vi "周期设置.vi"(11 "定时控制参数输入":T1) -> (3 "定时控制参数输出":T1)   [LabVIEW 2016, in "质控单元.lvlib"]
uses:
  <vilib>/Utility/miscctls.llb/LVPointTypeDef.ctl
panel:
  in  "采配水启用":bool
  in  "模块选择":T2
  in  "确定":bool
  in  "取消":bool
  in  "定时功能启用":bool
  out "选项卡控件":enum32{"定点启动", "间隔启动"}(tab)
  in  "24H周期设置":bool[](xcontrol)
  in  "已经启动次数":dbl
  in  "设定启动次数":dbl
  in  "定时间隔":dbl
  in  "周期设置类型":enum16{"定点启动", "间隔启动"}(ring)
  # "仪器测试类型："
  # "周期设置类型："
  # "请输入定时启动间隔"
  # "min"
  # "次"
  # "次"
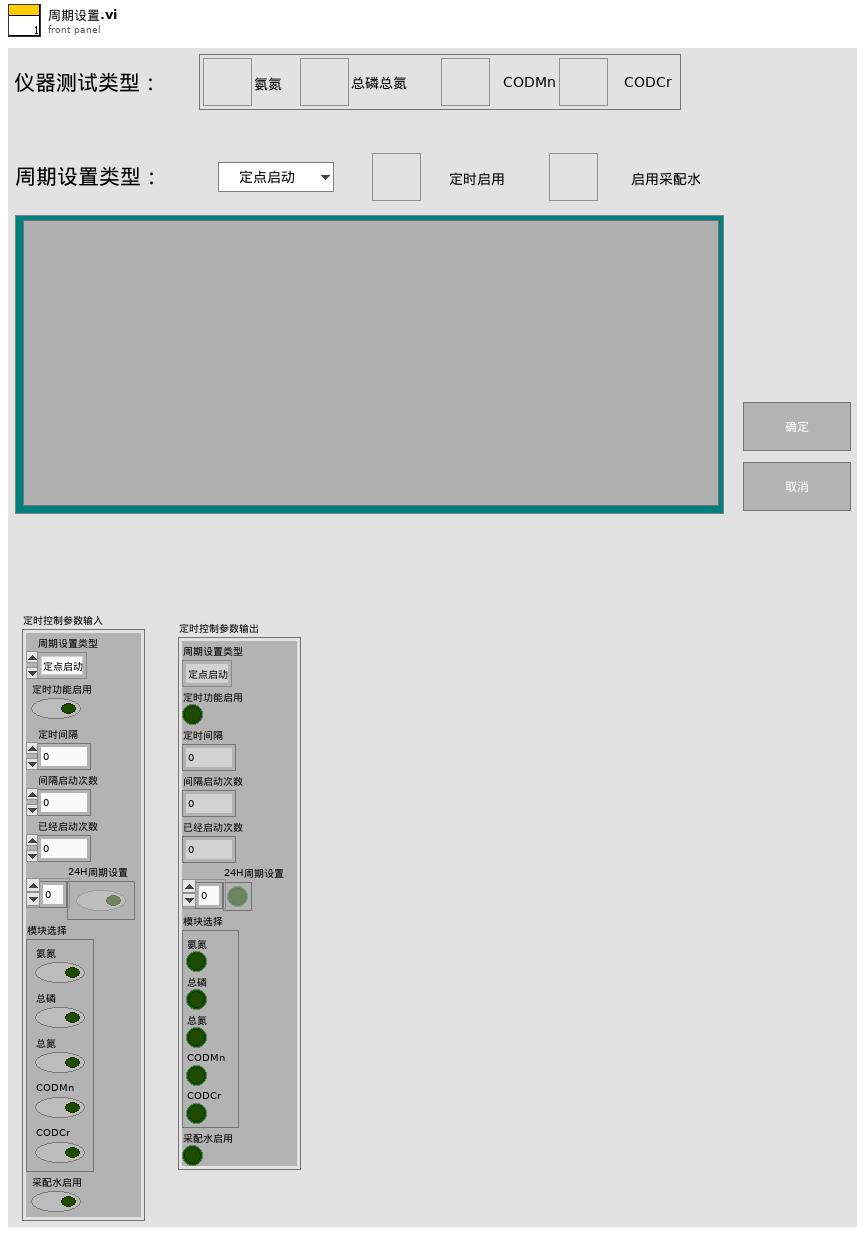
[diagram p1: front panel]
types:
  T1 = cluster{"周期设置类型":enum16{"定点启动", "间隔启动"}, "定时功能启用":bool, "定时间隔":dbl, "间隔启动次数":dbl, "已经启动次数":dbl, "24H周期设置":bool[], "模块选择":cluster{"氨氮":bool, "总磷":bool, "总氮":bool, "CODMn":bool, "CODCr":bool}, "采配水启用":bool}
  T2 = cluster{"氨氮":bool, "总磷":bool, "总氮":bool, "CODMn":bool, "CODCr":bool}
  T3 = typedef "LVPointTypeDef.ctl" = cluster{"Horizontal":i16, "Vertical":i16}
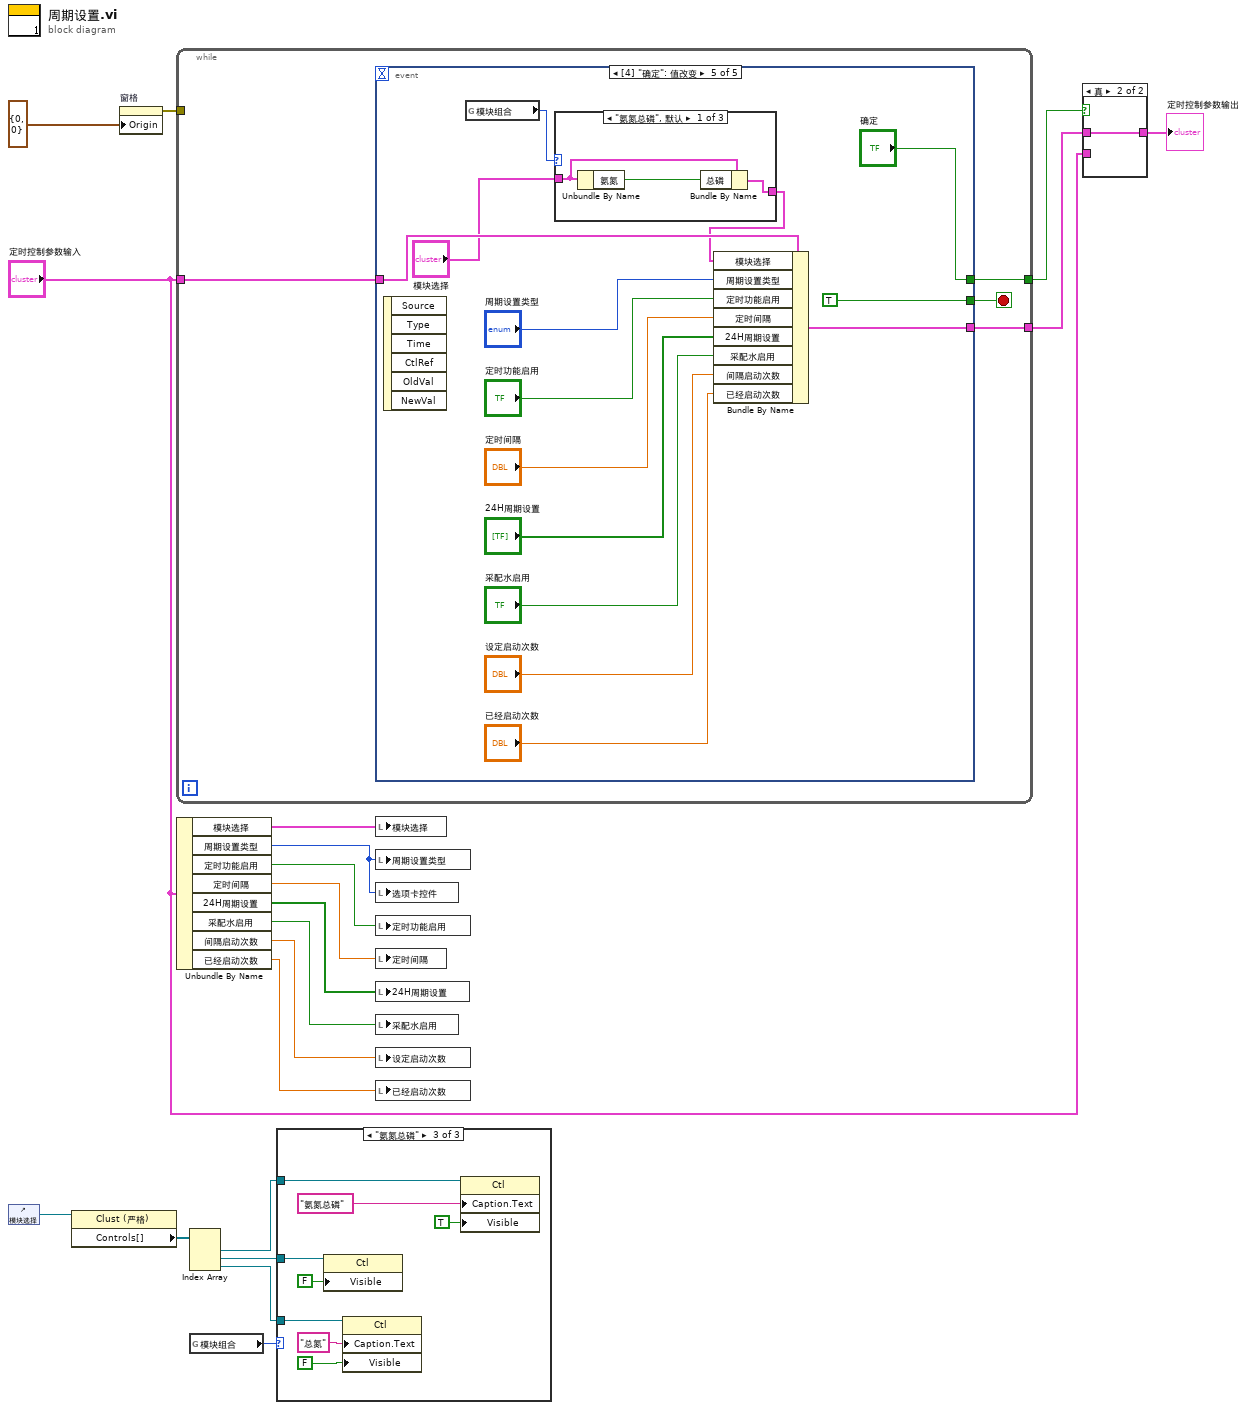
[diagram p0: block diagram]
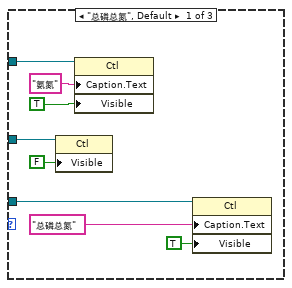
[diagram p2: hidden frame]
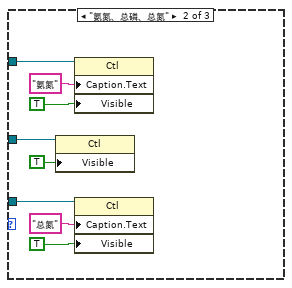
[diagram p3: hidden frame]
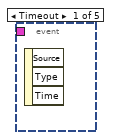
[diagram p5: hidden frame]
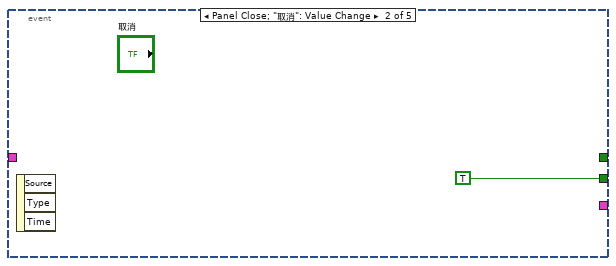
[diagram p6: hidden frame]
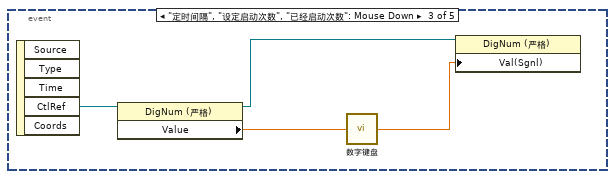
[diagram p7: hidden frame]
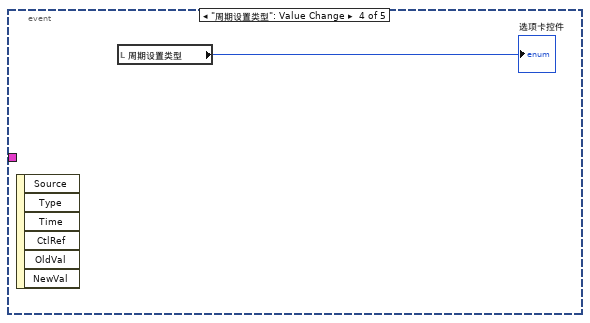
[diagram p8: hidden frame]
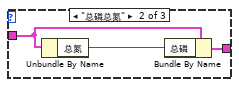
[diagram p9: hidden frame]
diagram:
  n1 = control-ref of="模块选择"() -> (w6:refnum<vi>)
  n2 = property class="Clust (严格)"(reference=w6) -> ("Controls[]"=w1:refnum<vi>[])  [unwired: 1 in, 2 out]
  n3 = property on="窗格" class="Pane"("Origin"=T3 {"Horizontal"=0, "Vertical"=0} ("原点")) -> (error out=w9:errorcluster)  [unwired: 2 in, 1 out]
  n4 = while {
    tunnel: [w23] -> w15
    tunnel: [w22] -> w16
    tunnel: "定时控制参数输入" -> [w21]
    tunnel: w9 -> [_]
    stop <- w24 stop-if-true
    n5 = event shown="[4] \"确定\": 值改变" {
      selector: _ -> [_ _ _ _ _]
      dyn-events: _ -> [_ _ _ _ _]
      timeout: _ -> [_ _ _ _ _]
      tunnel: [_ TRUE _ _ TRUE] -> w24
      tunnel: [_ _ _ _ w41] -> w23
      tunnel: [_ _ _ _ "确定"] -> w22
      tunnel: w21 -> [_ _ _ _ w37]
      event Timeout {
        n6 = event-data() -> ()  [unwired: 1 in, 3 out]
      }
      event Panel Close; "取消": Value Change {
        n7 = event-data() -> ()  [unwired: 1 in, 3 out]
      }
      event "定时间隔", "设定启动次数", "已经启动次数": Mouse Down {
        n8 = event-data() -> ("CtlRef"=w29:refnum<vi>)  [unwired: 1 in, 4 out]
        n9 = property class="DigNum (严格)"(reference=w29) -> (reference out=w26:refnum<vi>, "Value"=w28:dbl)  [unwired: 1 in, 1 out]
        n10 = call "数字键盘.vi"("OldNumber"=w28) -> ("NewNumber"=w27:sgl)
        n11 = property class="DigNum (严格)"(reference=w26, "Val(Sgnl)"=w27) -> ()  [unwired: 1 in, 2 out]
      }
      event "周期设置类型": Value Change {
        n12 = event-data() -> ()  [unwired: 1 in, 6 out]
        n13 = local read "周期设置类型"() -> (→"选项卡控件":enum16{"定点启动", "间隔启动"})
      }
      event "确定": Value Change {
        n14 = event-data() -> ()  [unwired: 1 in, 6 out]
        n15 = global read "断电保存全局.vi" "模块组合"() -> (w33:enum16{"氨氮总磷", "总磷总氮", "氨氮、总磷、总氮"})
        n16 = case shown="\"氨氮总磷\", 默认" w33 {
          tunnel: "模块选择" -> [w47 w49 w51]
          tunnel: [w45 w48 w51] -> w31
          frame "氨氮总磷", Default {
            n17 = Unbundle By Name(w47) -> ("氨氮"=w46:bool)
            n18 = Bundle By Name(cluster=w47, "总磷"=w46) -> (w45:T2)
          }
          frame "总磷总氮" {
            n19 = Unbundle By Name(w49) -> ("总氮"=w50:bool)
            n20 = Bundle By Name(cluster=w49, "总磷"=w50) -> (w48:T2)
          }
          frame "氨氮、总磷、总氮" {
          }
        }
        n21 = Bundle By Name(cluster=w37, "模块选择"=w31, "周期设置类型"="周期设置类型", "定时功能启用"="定时功能启用", "定时间隔"="定时间隔", "24H周期设置"="24H周期设置", "采配水启用"="采配水启用", "间隔启动次数"="设定启动次数", "已经启动次数"="已经启动次数") -> (w41:T1)
      }
    }
  }
  n22 = Unbundle By Name("定时控制参数输入") -> ("模块选择"=w14:T2, "周期设置类型"=w17:enum16{"定点启动", "间隔启动"}, "定时功能启用"=w20:bool, "定时间隔"=w19:dbl, "24H周期设置"=w18:bool[], "采配水启用"=w12:bool, "间隔启动次数"=w8:dbl, "已经启动次数"=w7:dbl)
  n23 = Index Array(array=w1) -> (element #1=w5:refnum<vi>, element #2=w4:refnum<vi>, element #3=w3:refnum<vi>)  [unwired: 3 in]
  n24 = global read "断电保存全局.vi" "模块组合"() -> (w2:enum16{"氨氮总磷", "总磷总氮", "氨氮、总磷、总氮"})
  n25 = case shown="\"氨氮总磷\"" w2 {
    tunnel: w5 -> [w59 w67 w75]
    tunnel: w4 -> [w57 w65 w73]
    tunnel: w3 -> [w54 w62 w70]
    frame "总磷总氮", Default {
      n26 = property class="Ctl"(reference=w57, "Visible"=FALSE ("可见")) -> ()  [unwired: 1 in, 2 out]
      n27 = property class="Ctl"(reference=w59, "Caption.Text"="氨氮" ("标题.文本"), "Visible"=TRUE ("可见")) -> ()  [unwired: 1 in, 2 out]
      n28 = property class="Ctl"(reference=w54, "Caption.Text"="总磷总氮" ("标题.文本"), "Visible"=TRUE ("可见")) -> ()  [unwired: 1 in, 2 out]
    }
    frame "氨氮、总磷、总氮" {
      n29 = property class="Ctl"(reference=w65, "Visible"=TRUE ("可见")) -> ()  [unwired: 1 in, 2 out]
      n30 = property class="Ctl"(reference=w67, "Caption.Text"="氨氮" ("标题.文本"), "Visible"=TRUE ("可见")) -> ()  [unwired: 1 in, 2 out]
      n31 = property class="Ctl"(reference=w62, "Caption.Text"="总氮" ("标题.文本"), "Visible"=TRUE ("可见")) -> ()  [unwired: 1 in, 2 out]
    }
    frame "氨氮总磷" {
      n32 = property class="Ctl"(reference=w73, "Visible"=FALSE ("可见")) -> ()  [unwired: 1 in, 2 out]
      n33 = property class="Ctl"(reference=w70, "Caption.Text"="总氮" ("标题.文本"), "Visible"=FALSE ("可见")) -> ()  [unwired: 1 in, 2 out]
      n34 = property class="Ctl"(reference=w75, "Caption.Text"="氨氮总磷" ("标题.文本"), "Visible"=TRUE ("可见")) -> ()  [unwired: 1 in, 2 out]
    }
  }
  n35 = local write "模块选择"(w14) -> ()
  n36 = local write "周期设置类型"(w17) -> ()
  n37 = local write "选项卡控件"(w17) -> ()
  n38 = local write "定时功能启用"(w20) -> ()
  n39 = local write "定时间隔"(w19) -> ()
  n40 = local write "24H周期设置"(w18) -> ()
  n41 = local write "采配水启用"(w12) -> ()
  n42 = local write "设定启动次数"(w8) -> ()
  n43 = local write "已经启动次数"(w7) -> ()
  n44 = case shown="真" w16 {
    tunnel: w15 -> [_ w77]
    tunnel: [w76 w77] -> w13
    tunnel: "定时控制参数输入" -> [w76 _]
    frame False {
    }
    frame True {
    }
  }
  "定时控制参数输出" <- w13
